vi "Read All owning libs.vi"(11 "SolutionBuilder in":refnum<class "SolutionBuilder.lvclass">) -> (2 "All owning libs":set{string}(c389), 3 "SolutionBuilder out":refnum<class "SolutionBuilder.lvclass">)   [LabVIEW 2020, in "SolutionBuilder.lvlib" / "SolutionBuilder.lvclass"]
uses:
  SolutionBuilder.lvclass
  ProjectItem/ProjectItem.lvclass
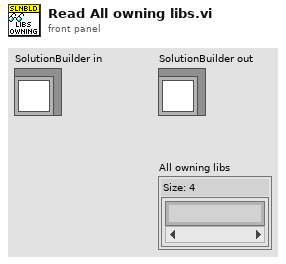
[diagram p1: front panel]
types:
  T1 = typedef "SolutionBuilder.lvlib/SolutionBuilder.lvclass/ProjectItemMap.ctl" = map{path, refnum<class "ProjectItem.lvclass">[]}
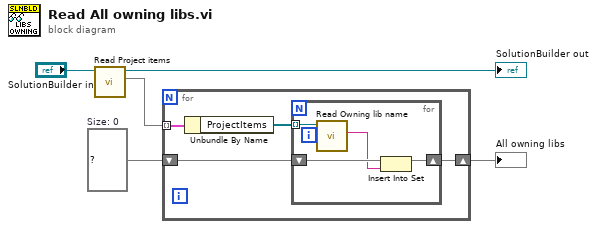
[diagram p0: block diagram]
diagram:
  w5 = set{string} {}  # Size: 0
  n1 = call-dynamic "Read Project items.vi"("SolutionBuilder in"="SolutionBuilder in") -> ("Project items"=w1:T1, "SolutionBuilder out"=→"SolutionBuilder out":refnum<class "SolutionBuilder.lvclass">)  [unwired: 9 in]
  n2 = for {
    tunnel: w1 -> [w9] mode=indexing
    shift-right: [w7] -> w4
    shift-left: w5 -> [w6]
    n3 = Unbundle By Name(w9) -> ("ProjectItems"=w8:refnum<class "ProjectItem.lvclass">[])
    n4 = for {
      tunnel: w8 -> [w11] mode=indexing
      shift-right: [w13] -> w7
      shift-left: w6 -> [w12]
      n5 = call-dynamic "Read Owning lib name.vi"("ProjectItem in"=w11) -> ("Owning lib name"=w10:string)  [unwired: 9 in, 1 out]
      n6 = Insert Into Set(10:w10, 11:w12) -> (3:w13:set{string})  [unwired: 1 out]
    }
  }
  "All owning libs" <- w4
